vi "CC GUI Recursive Load Folder to Tree.vi"(5 "Parent Tag":string, 7 "Tree Ref":refnum<vi>, 8 "error in (no error)":errorcluster, 9 "Depth":i32, 10 "Indent":i32, 11 "Path":path) -> (0 "error out":errorcluster)   [LabVIEW 2021]
panel:
  out "filenames":string[](array[string])
  out "name":string
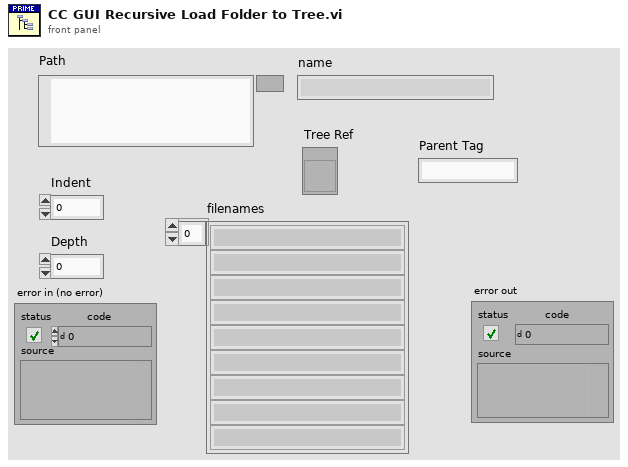
[diagram p1: front panel]
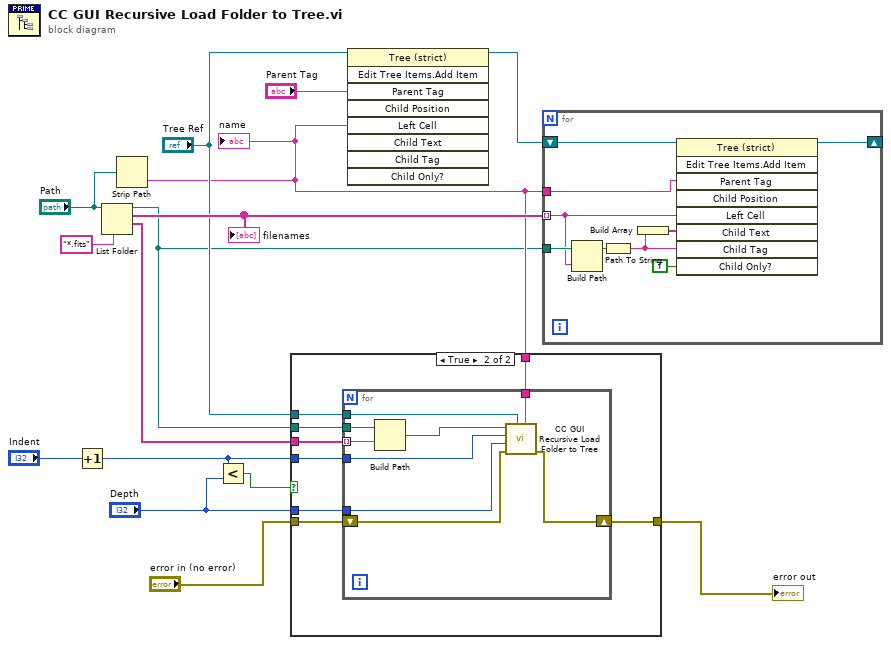
[diagram p0: block diagram]
diagram:
  n1 = Increment(x="Indent") -> (x+1=w8:i32)
  n2 = List Folder(path="Path", pattern="*.fits") -> (path out=w2:path, filenames=w14:string[], folder names=w13:string[])  [unwired: 2 in, 1 out]
  "filenames" <- w14
  n3 = Strip Path(path="Path") -> (name=w3:string)  [unwired: 1 out]
  "name" <- w3
  n4 = Less?(x=w8, y="Depth") -> (x < y?=w12:bool)
  n5 = case shown="True" w12 {
    tunnel: w2 -> [_ w24]
    tunnel: w13 -> [_ w23]
    tunnel: "Tree Ref" -> [_ w22]
    tunnel: w8 -> [_ w21]
    tunnel: "error in (no error)" -> [w16 w20]
    tunnel: [w16 w19] -> w10
    tunnel: "Depth" -> [_ w18]
    tunnel: w3 -> [_ w17]
    frame False {
    }
    frame True {
      n6 = for {
        tunnel: w24 -> [w33]
        tunnel: w23 -> [w32] mode=indexing
        tunnel: w21 -> [w31]
        tunnel: w22 -> [w29]
        shift-right: [w27] -> w19
        shift-left: w20 -> [w28]
        tunnel: w18 -> [w26]
        tunnel: w17 -> [w25]
        n7 = Build Path(base path=w33, name or relative path=w32) -> (appended path=w30:path)
        n8 = call "CC GUI Recursive Load Folder to Tree.vi"("Parent Tag"=w25, "Tree Ref"=w29, "error in (no error)"=w28, "Depth"=w26, "Indent"=w31, "Path"=w30) -> ("error out"=w27:errorcluster)  [unwired: 5 in]
      }
    }
  }
  "error out" <- w10
  n9 = invoke on="Invoke Node" class="Tree (strict)" method="Edit Tree Items.Add Item"(reference="Tree Ref", "Parent Tag"="Parent Tag", "Left Cell"=w3) -> (reference out=w6:refnum<vi>)  [unwired: 6 in, 8 out]
  n10 = for {
    tunnel: w14 -> [w36] mode=indexing
    shift-right: [w41] -> _
    shift-left: w6 -> [w42]
    tunnel: w3 -> [w40]
    tunnel: w2 -> [w37]
    n11 = Build Path(base path=w37, name or relative path=w36) -> (appended path=w35:path)
    n12 = Path To String(path=w35) -> (string=w39:string)
    n13 = Build Array(w39) -> (w38:string[])
    n14 = invoke on="Invoke Node" class="Tree (strict)" method="Edit Tree Items.Add Item"(reference=w42, "Parent Tag"=w40, "Left Cell"=w36, "Child Text"=w38, "Child Tag"=w39, "Child Only?"=TRUE) -> (reference out=w41:refnum<vi>)  [unwired: 3 in, 8 out]
  }
